vi "Format Sample To Time.vi"(11 "Samples":i32) -> (3 "Formatted Time":string)   [LabVIEW 2018, in "User Interface.lvlib"]
doc: "Convert the sample number into a time value in the form HH:MM:SS.s"
uses:
  User Interface.lvlib
  Globals/Constants.vi
  Globals/Globals.lvlib
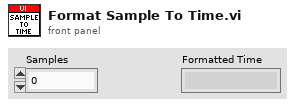
[diagram p1: front panel]
types:
  T1 = typedef "LVDateTimeRec.ctl" = cluster{"fractional second":dbl, "second":i32, "minute":i32, "hour":i32, "day of month":i32, "month":i32, "year":i32, "day of week":i32, "day of year":i32, "DST":i32}
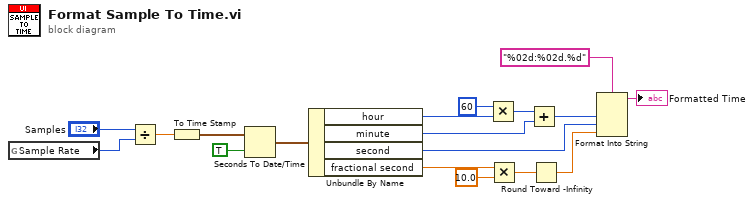
[diagram p0: block diagram]
diagram:
  n1 = global read "Constants.vi" "Sample Rate"() -> (w1:i32)
  n2 = Divide(x="Samples", y=w1) -> (x/y=w17:dbl)
  n3 = To Time Stamp(1:w17) -> (0:w16:timestamp)
  n4 = Seconds To Date/Time(time stamp (now)=w16, to UTC (F)=TRUE) -> (date time rec=w14:T1)
  n5 = Unbundle By Name(w14) -> ("hour"=w12:i32, "minute"=w9:i32, "second"=w7:i32, "fractional second"=w6:dbl)
  n6 = Multiply(x=60, y=w12) -> (x*y=w10:i32)
  n7 = Multiply(x=w6, y=10.0) -> (x*y=w4:dbl)
  n8 = Add(x=w10, y=w9) -> (x+y=w8:i32)
  n9 = Round Toward -Infinity(1:w4) -> (0:w3:dbl)
  n10 = Format Into String(format string="%02d:%02d.%d", w8, w7, w3) -> (resulting string=→"Formatted Time":string)  [unwired: 2 in, 1 out]
